vi "Configure Horizontal Timing.vi"(8 "error in":errorcluster, 11 "FPGA Session":T1) -> (0 "error out":errorcluster, 3 "FPGA Session":T1)   [LabVIEW 2011]
uses:
  <userlib>/FlexRIO Host Library/FlexRIO Host API/Session/FPGA Session Ref.ctl
  <userlib>/FlexRIO Host Library/FlexRIO Host Library (User).lvlib
panel:
  in  "Record Count":u16=1
  in  "% of Hold Off Time":dbl=10.0
  in  "% of Pre-Trigger Samples":dbl=10.0
  in  "Record Length":u16=30
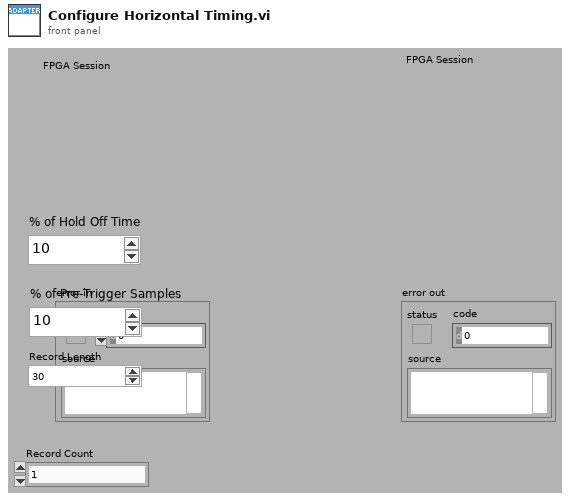
[diagram p1: front panel]
types:
  T1 = typedef "FlexRIO Host Library (User).lvlib/FPGA Session Ref.ctl" = refnum<k20>
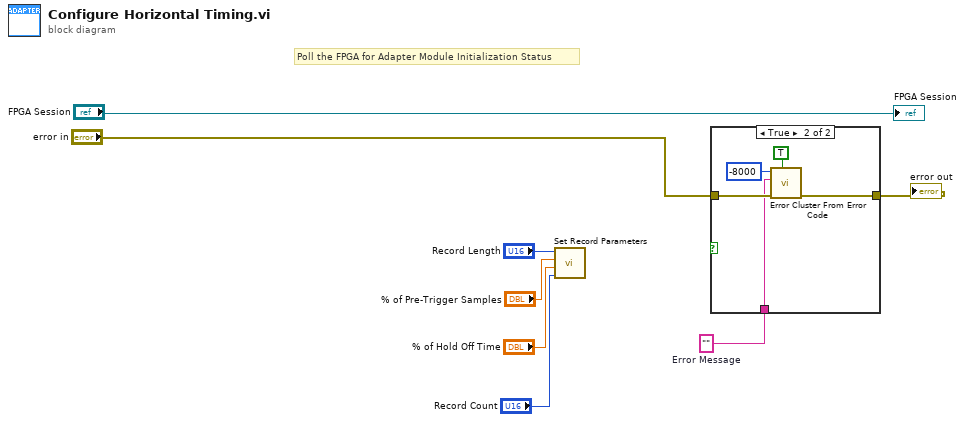
[diagram p0: block diagram]
diagram:
  w6 = ""  # Error Message
  # "Poll the FPGA for Adapter Module Initialization Status"
  n1 = call <userlib>:"Set Record Parameters.vi"("Record Count"="Record Count", "% of Hold Off Time"="% of Hold Off Time", "% of Pre-Trigger Samples"="% of Pre-Trigger Samples", "Total Number of Samples"="Record Length") -> ()  [unwired: 4 in, 4 out]
  n2 = case shown="True" {
    selector: _ -> [_ _]
    tunnel: "error in" -> [w9 w13]
    tunnel: [w9 w12] -> w7
    tunnel: w6 -> [_ w11]
    frame False {
    }
    frame True {
      n3 = call <vilib>:"Error Cluster From Error Code.vi"("show call chain? (False)"=TRUE, "error in (no error)"=w13, "error message (\"\")"=w11, "error code (0)"=-8000) -> ("error out"=w12:errorcluster)  [unwired: 5 in]
    }
  }
  "error out" <- w7
  "FPGA Session" <- "FPGA Session"
